vi "Simulation Record Write.vi"(8 "Error In":errorcluster, 11 "simulator":T1={"configuration"={"maxTime"=5.0, "enableVisualization"=TRUE, "Environment Definition"=path "iRobot Navigation State Machine.vi", "Record Location"=path "Simulation Record.xml", "autograde?"=TRUE, "interactive?"=FALSE, "Feedback Mode"=enum."debug navigation", "Robot State Charts"=[path "C:/Users/blueuser/Desktop/Robo Sim Berkley/cpsgrader-release-0.4/Simulators/EECS149lab/src/LabVIEW/statechart/Simulation Statechart.vi"], "statechart"=path "C:/Users/blueuser/Desktop/Robo Sim Berkley/cpsgrader-release-0.4/Simulators/EECS149lab/src/LabVIEW/statechart/Simulation Statechart.vi"}, "Statechart\ndisplay"=refnum, "first step?"=FALSE, "Robots Simulation Statecharts"=[], "Robots"=[]}) -> (0 "Error Out":errorcluster, 3 "simulator":T1={"configuration"={"maxTime"=5.0, "enableVisualization"=TRUE, "Environment Definition"=path "iRobot Navigation State Machine.vi", "Record Location"=path "Simulation Record.xml", "autograde?"=TRUE, "interactive?"=FALSE, "Feedback Mode"=enum."debug navigation", "Robot State Charts"=[path "C:/Users/blueuser/Desktop/Robo Sim Berkley/cpsgrader-release-0.4/Simulators/EECS149lab/src/LabVIEW/statechart/Simulation Statechart.vi"], "statechart"=path "C:/Users/blueuser/Desktop/Robo Sim Berkley/cpsgrader-release-0.4/Simulators/EECS149lab/src/LabVIEW/statechart/Simulation Statechart.vi"}, "Statechart\ndisplay"=refnum, "first step?"=FALSE, "Robots Simulation Statecharts"=[], "Robots"=[]})   [LabVIEW 2015]
uses:
  Simulator.ctl
  CyberSim interface/Simulation Configuration.ctl
  autograder/feedbackMode.ctl
  Multi Bot Code/RobotData.ctl
  <instrlib>/DC Motor Controller/HAIOL/DC Motor Controller.lvclass
  <vilib>/Utility/xml.llb/Write to XML File(string).vi
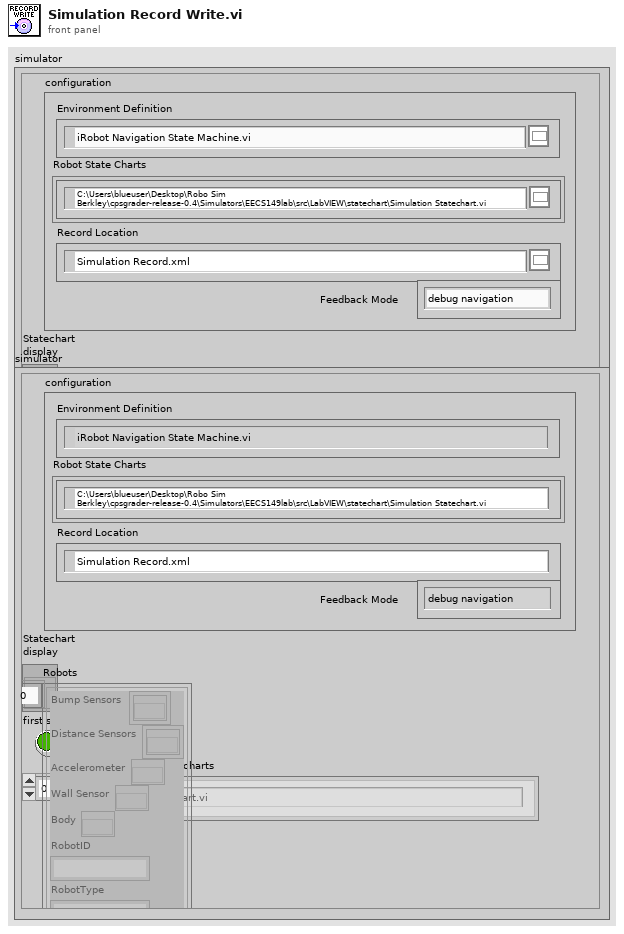
[diagram p1: front panel]
types:
  T1 = typedef "Simulator.ctl" = cluster{"configuration":T2, "Statechart\ndisplay":refnum<vi>, "first step?":bool, "Robots Simulation Statecharts":path[], "Robots":T4[]}
  T2 = typedef "Simulation Configuration.ctl" = cluster{"maxTime":sgl, "enableVisualization":bool, "Environment Definition":path, "Record Location":path, "autograde?":bool, "interactive?":bool, "Feedback Mode":T3, "Robot State Charts":path[], "statechart":path}
  T3 = typedef "feedbackMode.ctl" = enum32{"debug navigation", "debug hill climb", "autograde navigation", "autograde hill climb"}
  T4 = typedef "RobotData.ctl" = cluster{"Bump Sensors":refnum<k20>[], "Distance Sensors":refnum<k20>[], "Accelerometer":refnum<k20>, "Wall Sensor":refnum<k20>, "Body":refnum<k20>, "RobotID":string, "RobotType":string, "Left Motor":refnum<class "DC Motor Controller.lvclass">, "Right Motor":refnum<class "DC Motor Controller.lvclass">}
  T5 = typedef "Simulation Record.ctl" = cluster{"configuration":T2, "trace":T6[], "environment MD5":string, "statechart MD5":string, "record timestamp":string}
  T6 = typedef "Simulation Trace Element.ctl" = cluster{"sensors":T7, "position":T12, "orientation":T13, "Simulation Time (s)":sgl}
  T7 = typedef "Sensors.ctl" = cluster{"net distance (mm)":i32, "net angle (deg)":i32, "accelerometer":T8, "Is Simulator?":bool, "Kobuki Sensors":T9, "Requested Left Wheel Velocity(mm/s)":i32, "Requested Right Wheel Velocity(mm/s)":i32}
  T8 = typedef "Accelerometer.ctl" = cluster{"x axis (g)":dbl, "y axis (g)":dbl, "z axis (g)":dbl}
  T9 = typedef "KobukiSensors.ctl" = cluster{"Bumps + Wheel Drops":T10, "Cliff Left":bool, "Cliff Center":bool, "Cliff Right":bool, "Cliff Left Signal":u16, "Cliff Center Signal":u16, "Cliff Right Signal":u16, "Buttons":T11, "Left Wheel Encoder (ticks)":u16, "Right Wheel Encoder (ticks) ":u16, "Left  Wheel PWM":i8, "Right Wheel PWM":i8, "Left Wheel OverCurrent":bool, "Right Wheel OverCurrent ":bool, "Right Wheel Current (x10mA)":i16, "Left  Wheel Current  (x10mA)":i16, "TimeStamp":u16, "Battery Voltage (mV)":i16, "Angle( of 100deg)":i16, "Angle Rate( of 100 deg/sec)":i16, "Charger Source ":i8}
  T10 = typedef "Kobuki Bumps and WheelDrops.ctl" = cluster{"Wheeldrop Left":bool, "Wheeldrop Right":bool, "Bump Left":bool, "Bump Center":bool, "Bump Right":bool}
  T11 = typedef "Kobuki Buttons.ctl" = cluster{"B0":bool, "B1":bool, "B2":bool}
  T12 = typedef "Simulated Position.ctl" = cluster{"x (m)":sgl, "y (m)":sgl, "z (m)":sgl}
  T13 = typedef "Simulated Orientation.ctl" = cluster{"roll (deg)":sgl, "pitch (deg)":sgl, "yaw (deg)":sgl}
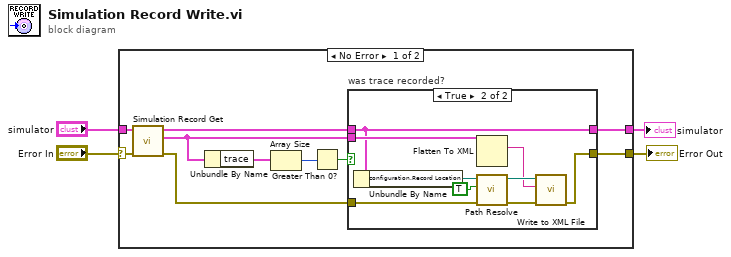
[diagram p0: block diagram]
diagram:
  n1 = case shown="No Error" "Error In" {
    selector: "Error In" -> [w5 w26]
    tunnel: [w14 w26] -> w4
    tunnel: "simulator" -> [w13 w27]
    tunnel: [w6 w27] -> w2
    frame No Error {
      n2 = call "Simulation Record Get.vi"("Error In"=w5, "simulator"=w13) -> ("Error Out"=w11:errorcluster, "record"=w10:T5, "simulator"=w12:T1)  [unwired: 7 in]
      n3 = Unbundle By Name(w10) -> ("trace"=w9:T6[])
      n4 = Array Size(array=w9) -> (size(s)=w8:i32)
      n5 = Greater Than 0?(x=w8) -> (x > 0?=w7:bool)
      n6 = case "was trace recorded?" shown="True" w7 {
        tunnel: [w16 w25] -> w14
        tunnel: w12 -> [w15 w17]
        tunnel: w11 -> [w16 w19]
        tunnel: w10 -> [_ w18]
        tunnel: [w15 w17] -> w6
        frame False {
        }
        frame True {
          n7 = Unbundle By Name(w17) -> ("configuration.Record Location"=w20:path)
          n8 = Flatten To XML(anything=w18) -> (xml string=w21:string)
          n9 = call "Path Resolve.vi"("Error In"=w19, "create?"=TRUE, "absolute or relative path"=w20) -> ("Error Out"=w22:errorcluster, "resolved path"=w23:path)  [unwired: 7 in]
          n10 = call-poly <vilib>:"Write to XML File.vi"("error in (no error)"=w22, "XML Input"=w21, "XML File Path"=w23) -> ("error out"=w25:errorcluster)  [unwired: 6 in, 2 out]
        }
      }
    }
    frame Error {
    }
  }
  "Error Out" <- w4
  "simulator" <- w2
